vi "test Init Close.vi"(11 "Test Case In":refnum<class "Test Cases.lvclass">) -> (0 "error out":errorcluster, 3 "Test Case Out":refnum<class "Test Cases.lvclass">)   [LabVIEW 2024, in "Test Cases.lvclass"]
uses:
  Test Cases.lvclass
  MyTestHeader/MyTestHeader.lvclass
  source/Grid/SourceGrid.lvclass
  source/System.Drawing.Color.ctl
  <vilib>/Astemes/LUnit/Test Case.lvclass/Test Case.ctl
  <vilib>/Astemes/LUnit/Append Pass Result.vi
  <vilib>/Astemes/LUnit/Append Fail Result.vi
  <vilib>/Astemes/LUnit/Run In UI.vi
  <vilib>/Utility/error.llb/Clear Errors.vi
  source/Grid/Set FixedRows.vi
  source/Grid/Set SelectionMode.vi
  <vilib>/Astemes/LUnit/Test Case.lvclass
  source/SourceGrid.lvlib
  D:/git/Sourcegrid-LabVIEW/dll/SourceGrid.dll
  dll/SourceGrid.dll
panel:
  in  "Grid Container":refnum<k24>(container)
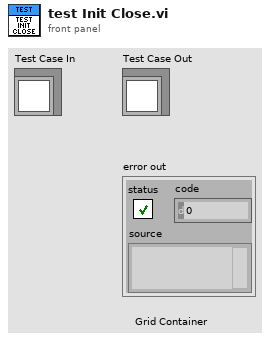
[diagram p1: front panel]
types:
  T1 = typedef "SourceGrid.lvlib/System.Drawing.Color.ctl" = enum16{"AliceBlue", "AntiqueWhite", "Aqua", "Aquamarine", "Azure", "Beige", "Bisque", "Black", "BlanchedAlmond", "Blue", "BlueViolet", "Brown", "BurlyWood", "CadetBlue", "Chartreuse", "Chocolate", "Coral", "CornflowerBlue", "Cornsilk", "Crimson", "Cyan", "DarkBlue", "DarkCyan", "DarkGoldenrod", "DarkGray", "DarkGreen", "DarkKhaki", "DarkMagenta", "DarkOliveGreen", "DarkOrange", "DarkOrchid", "DarkRed", "DarkSalmon", "DarkSeaGreen", "DarkSlateBlue", "DarkSlateGray", "DarkTurquoise", "DarkViolet", "DeepPink", "DeepSkyBlue", "DimGray", "DodgerBlue", "Firebrick", "FloralWhite", "ForestGreen", "Fuchsia", "Gainsboro", "GhostWhite", "Gold", "Goldenrod", "Gray", "Green", "GreenYellow", "Honeydew", "HotPink", "IndianRed", "Indigo", "Ivory", "Khaki", "Lavender", "LavenderBlush", "LawnGreen", "LemonChiffon", "LightBlue", "LightCoral", "LightCyan", "LightGoldenrodYellow", "LightGray", "LightGreen", "LightPink", "LightSalmon", "LightSeaGreen", "LightSkyBlue", "LightSlateGray", "LightSteelBlue", "LightYellow", "Lime", "LimeGreen", "Linen", "Magenta", "Maroon", "MediumAquamarine", "MediumBlue", "MediumOrchid", "MediumPurple", "MediumSeaGreen", "MediumSlateBlue", "MediumSpringGreen", "MediumTurquoise", "MediumVioletRed", "MidnightBlue", "MintCream", "MistyRose", "Moccasin", "NavajoWhite", "Navy", "OldLace", "Olive", "OliveDrab", "Orange", "OrangeRed", "Orchid", "PaleGoldenrod", "PaleGreen", "PaleTurquoise", "PaleVioletRed", "PapayaWhip", "PeachPuff", "Peru", "Pink", "Plum", "PowderBlue", "Purple", "Red", "RosyBrown", "RoyalBlue", "SaddleBrown", "Salmon", "SandyBrown", "SeaGreen", "SeaShell", "Sienna", "Silver", "SkyBlue", "SlateBlue", "SlateGray", "Snow", "SpringGreen", "SteelBlue", "Tan", "Teal", "Thistle", "Tomato", "Transparent", "Turquoise", "Violet", "Wheat", "White", "WhiteSmoke", "Yellow"}
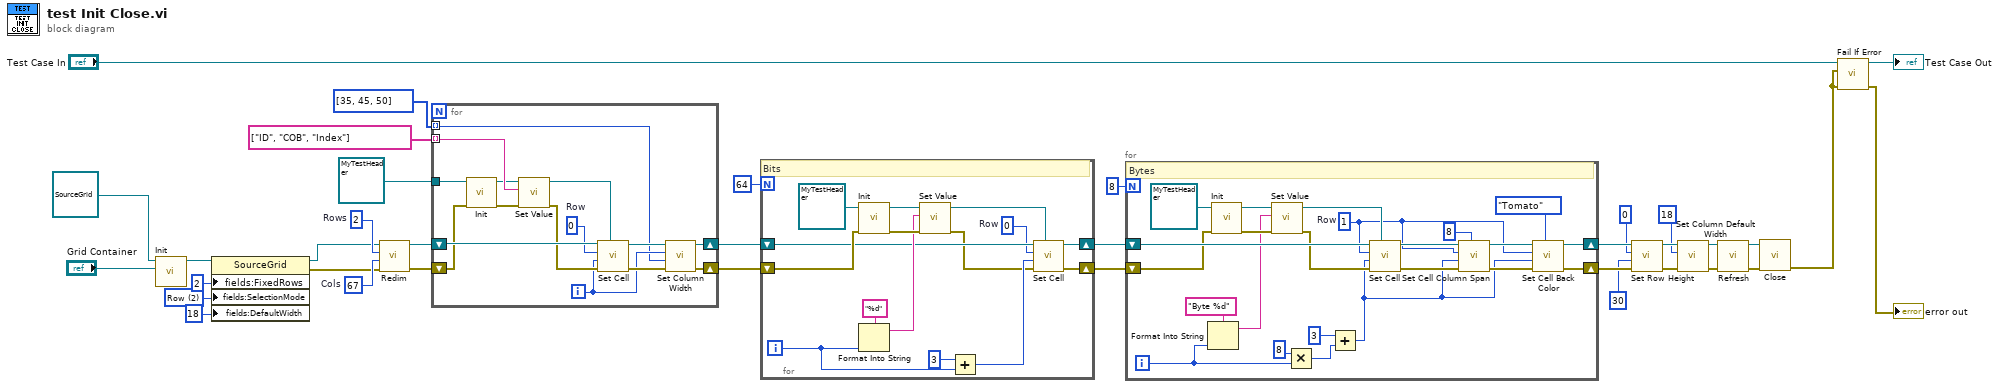
[diagram p0: block diagram]
diagram:
  w30 = 2 items=["Cell"=1, "Row"=2, "Column"=3] ("SelectionMode")
  w31 = 67  # Cols
  w32 = 2  # Rows
  n1 = call-dynamic "Init.vi"("Sourcegrid Container"="Grid Container", "Grid in"=refnum<class "SourceGrid.lvclass"> refnum) -> ("Grid out"=w9:refnum<class "SourceGrid.lvclass">)  [unwired: 8 in, 1 out]
  n2 = property class="SourceGrid"(reference=w9, "fields:FixedRows"=2 ("FixedRows"), "fields:SelectionMode"=w30, "fields:DefaultWidth"=18 ("DefaultWidth")) -> (reference out=w8:refnum<class "SourceGrid.lvclass">, error out=w6:errorcluster)  [unwired: 1 in]
  n3 = call "Redim.vi"("error in"=w6, "Columns"=w31, "Rows"=w32, "Sourcegrid in"=w8) -> ("error out"=w5:errorcluster, "Sourcegrid out"=w7:refnum<class "SourceGrid.lvclass">)  [unwired: 6 in]
  n4 = for {
    shift-right: [w45] -> w22
    shift-left: w5 -> [w48]
    shift-right: [w43] -> w23
    shift-left: w7 -> [w51]
    tunnel: string[] ["ID", "COB", "Index"] -> [w40] mode=indexing
    tunnel: refnum<class "MyTestHeader.lvclass"> refnum ("MyTestHeader.lvclass") -> [w38]
    tunnel: i32[] [35, 45, 50] -> [w41] mode=indexing
    i -> [w42]
    w49 = 0  # Row
    n5 = call-dynamic "Init.vi"("error in"=w48, "MyTestHeader in"=w38) -> ("error out"=w39:errorcluster, "MyTestHeader out"=w37:refnum<class "MyTestHeader.lvclass">)  [unwired: 8 in]
    n6 = call-dynamic "Set Value.vi"("error in"=w39, "Value"=w40, "MyTestHeader in"=w37) -> ("error out"=w46:errorcluster, "MyTestHeader out"=w47:refnum<class "MyTestHeader.lvclass">)  [unwired: 7 in]
    n7 = call "Set Cell.vi"("Cell"=w47, "error in"=w46, "Column"=w42, "Row"=w49, "Sourcegrid in"=w51) -> ("error out"=w50:errorcluster, "Sourcegrid out"=w44:refnum<class "SourceGrid.lvclass">)  [unwired: 5 in]
    n8 = call "Set Column Width.vi"("error in"=w50, "Width"=w41, "Column"=w42, "Sourcegrid in"=w44) -> ("error out"=w45:errorcluster, "Sourcegrid out"=w43:refnum<class "SourceGrid.lvclass">)  [unwired: 6 in]
  }
  n9 = for {
    N: 64 -> [_]
    shift-right: [w58] -> w19
    shift-left: w22 -> [w64]
    shift-right: [w57] -> w20
    shift-left: w23 -> [w56]
    i -> [w59]
    w55 = 0  # Row
    # "Bits"
    n10 = call-dynamic "Init.vi"("error in"=w64, "MyTestHeader in"=refnum<class "MyTestHeader.lvclass"> refnum ("MyTestHeader.lvclass")) -> ("error out"=w63:errorcluster, "MyTestHeader out"=w62:refnum<class "MyTestHeader.lvclass">)  [unwired: 8 in]
    n11 = Format Into String(format string="%d", w59) -> (resulting string=w61:string)  [unwired: 2 in, 1 out]
    n12 = call-dynamic "Set Value.vi"("error in"=w63, "Value"=w61, "MyTestHeader in"=w62) -> ("error out"=w53:errorcluster, "MyTestHeader out"=w52:refnum<class "MyTestHeader.lvclass">)  [unwired: 7 in]
    n13 = Add(x=3, y=w59) -> (x+y=w54:i32)
    n14 = call "Set Cell.vi"("Cell"=w52, "error in"=w53, "Column"=w54, "Row"=w55, "Sourcegrid in"=w56) -> ("error out"=w58:errorcluster, "Sourcegrid out"=w57:refnum<class "SourceGrid.lvclass">)  [unwired: 5 in]
  }
  n15 = for {
    N: 8 -> [_]
    shift-right: [w73] -> w18
    shift-left: w19 -> [w83]
    shift-right: [w71] -> w15
    shift-left: w20 -> [w88]
    i -> [w79]
    w69 = 1  # Row
    # "Bytes"
    n16 = Format Into String(format string="Byte %d", w79) -> (resulting string=w77:string)  [unwired: 2 in, 1 out]
    n17 = call-dynamic "Init.vi"("error in"=w83, "MyTestHeader in"=refnum<class "MyTestHeader.lvclass"> refnum ("MyTestHeader.lvclass")) -> ("error out"=w82:errorcluster, "MyTestHeader out"=w86:refnum<class "MyTestHeader.lvclass">)  [unwired: 8 in]
    n18 = call-dynamic "Set Value.vi"("error in"=w82, "Value"=w77, "MyTestHeader in"=w86) -> ("error out"=w81:errorcluster, "MyTestHeader out"=w84:refnum<class "MyTestHeader.lvclass">)  [unwired: 7 in]
    n19 = Multiply(x=8, y=w79) -> (x*y=w76:i32)
    n20 = Add(x=3, y=w76) -> (x+y=w68:i32)
    n21 = call "Set Cell.vi"("Cell"=w84, "error in"=w81, "Column"=w68, "Row"=w69, "Sourcegrid in"=w88) -> ("error out"=w89:errorcluster, "Sourcegrid out"=w75:refnum<class "SourceGrid.lvclass">)  [unwired: 5 in]
    n22 = call "Set Cell Column Span.vi"("Range"=8, "error in"=w89, "Column"=w68, "Row"=w69, "SourceGrid in"=w75) -> ("error out"=w70:errorcluster, "SourceGrid out"=w72:refnum<class "SourceGrid.lvclass">)  [unwired: 5 in]
    n23 = call "Set Cell Back Color.vi"("Color"=System.Drawing.Color."Tomato", "error in"=w70, "Column"=w68, "Row"=w69, "SourceGrid in"=w72) -> ("error out"=w73:errorcluster, "SourceGrid out"=w71:refnum<class "SourceGrid.lvclass">)  [unwired: 5 in]
  }
  n24 = call "Set Row Height.vi"("error in"=w18, "Height"=30, "Row"=0, "SourceGrid in"=w15) -> ("error out"=w16:errorcluster, "SourceGrid out"=w11:refnum<class "SourceGrid.lvclass">)  [unwired: 6 in]
  n25 = call "Set Column Default Width.vi"("error in"=w16, "Default Width"=18, "SourceGrid in"=w11) -> ("error out"=w24:errorcluster, "SourceGrid out"=w2:refnum<class "SourceGrid.lvclass">)  [unwired: 7 in]
  n26 = call "Refresh.vi"("error in"=w24, "SourceGrid in"=w2) -> ("error out"=w3:errorcluster, "SourceGrid out"=w1:refnum<class "SourceGrid.lvclass">)  [unwired: 8 in]
  n27 = call-dynamic "Close.vi"("error in"=w3, "Sourcegrid in"=w1) -> ("error out"=w27:errorcluster)  [unwired: 8 in, 1 out]
  n28 = call <vilib>:"Fail If Error.vi"("error in (no error)"=w27, "Assert error"=w27, "LUnit Test Case In"="Test Case In") -> ("error out"=→"error out":errorcluster, "LUnit Test Case Out"=→"Test Case Out":refnum<class "Test Cases.lvclass">)  [unwired: 7 in]
